vi "labview-traffic-light.vi"() -> ()   [LabVIEW 2022 SP3]
panel:
  out "Time":dbl
  in  "Yellow Time":dbl
  in  "Red Time":dbl
  in  "Green Time":dbl
  out "Red":bool
  out "yellow":bool
  out "Green":bool
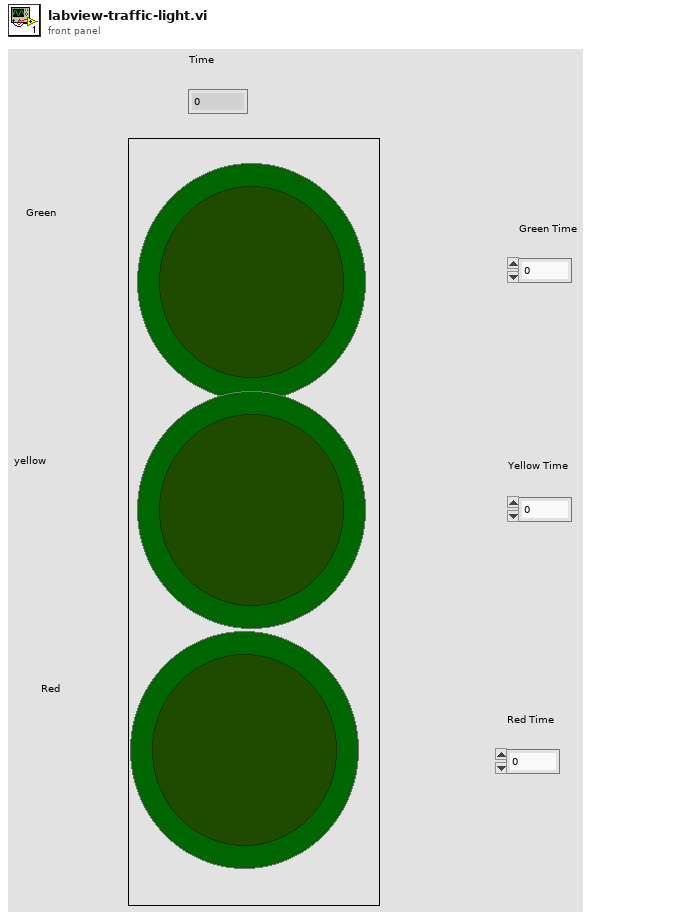
[diagram p1: front panel]
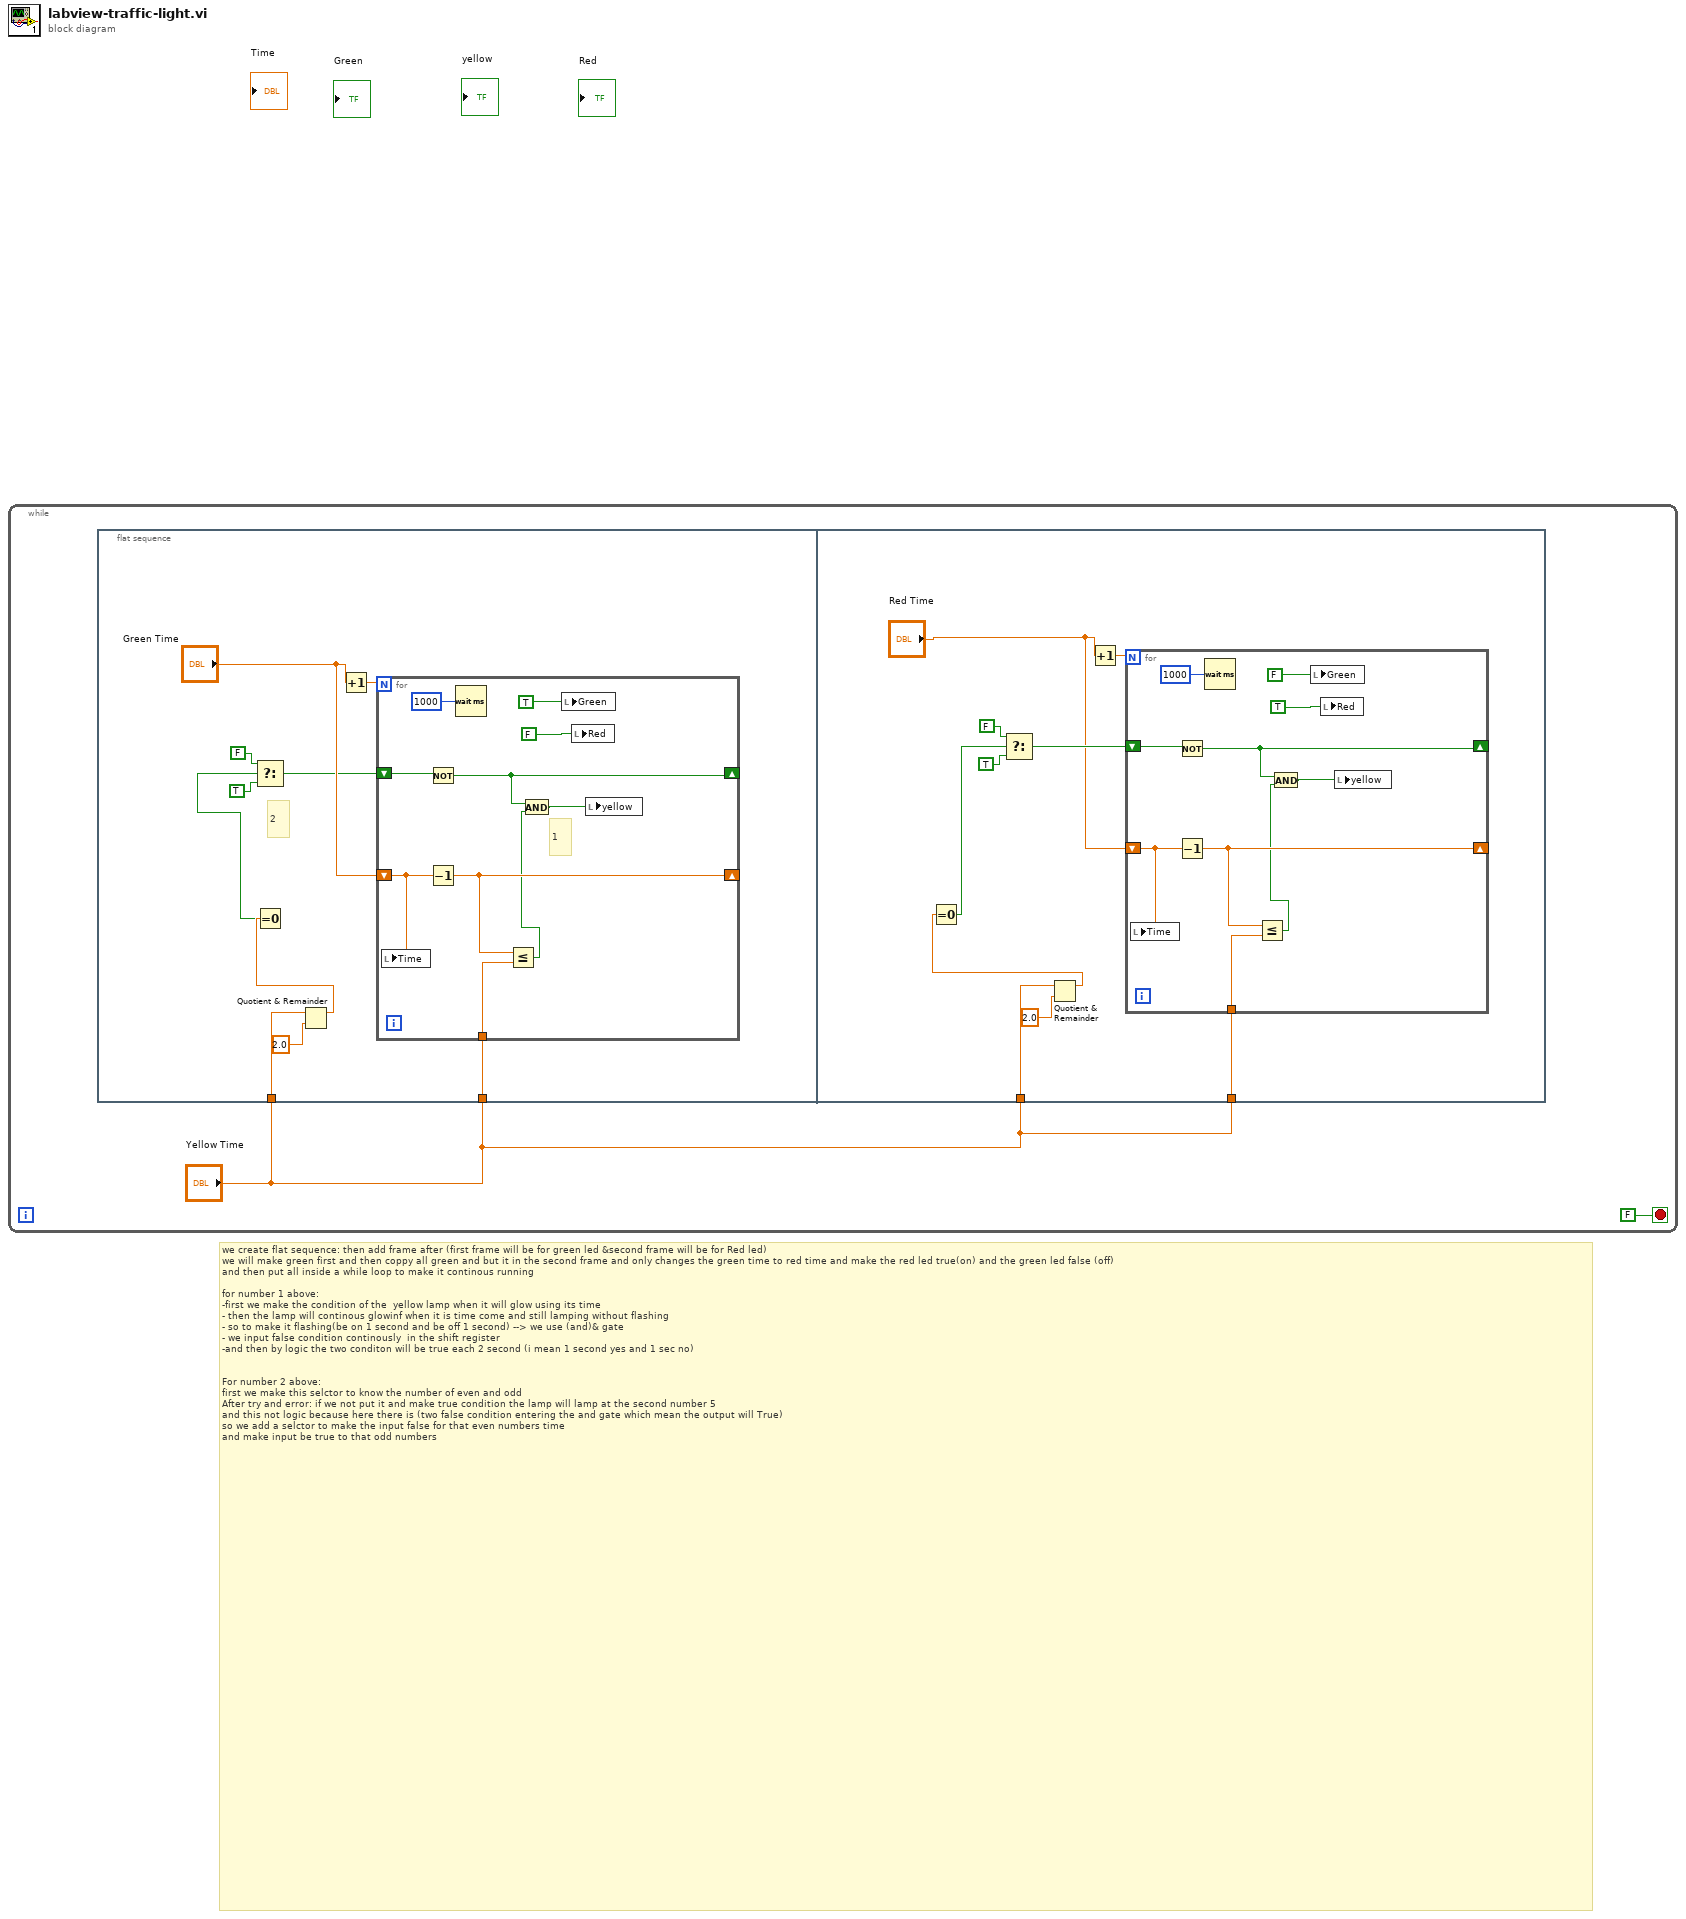
[diagram p0: block diagram]
diagram:
  # "we create flat sequence: then add frame after (first frame will be for green led &second frame will be for Red led)\nwe will make green first and then coppy all green and but it in the second frame and only changes the green time to red time and make the red led true(on) and the green led false (off) \nand then put all inside a while loop to make it continous running\n\nfor number 1 above:\n-first we make the condition of the  yellow lamp when it will glow using its time \n- then the lamp will continous glowinf when it is time come and still lamping without flashing\n- so to make it flashing(be on 1 second and be off 1 second) --> we use (and)& gate\n- we input false condition continously  in the shift register\n-and then by logic the two conditon will be true each 2 second (i mean 1 second yes and 1 sec no) \n\n\nFor number 2 above:\nfirst we make this selctor to know the number of even and odd\nAfter try and error: if we not put it and make true condition the lamp will lamp at the second number 5\nand this not logic because here there is (two false condition entering the and gate which mean the output will True)\nso we add a selctor to make the input false for that even numbers time \nand make input be true to that odd numbers"
  n1 = while {
    stop <- FALSE stop-if-true
    n2 = flat-sequence {
      tunnel: "Yellow Time" -> [w12]
      tunnel: "Yellow Time" -> [w8]
      tunnel: "Yellow Time" -> [w26]
      tunnel: "Yellow Time" -> [w25]
      frame #0 {
        # "2"
        n3 = Quotient & Remainder(x=w8, y=2.0) -> (x-y*floor(x/y)=w6:dbl)  [unwired: 1 out]
        n4 = Equal To 0?(x=w6) -> (x = 0?=w5:bool)
        n5 = Select(t=FALSE, s=w5, f=TRUE) -> (s? t:f=w9:bool)
        n6 = Increment(x="Green Time") -> (x+1=w11:dbl)
        n7 = for {
          N: w11 -> [_]
          shift-right: [w17] -> _
          shift-left: "Green Time" -> [w19]
          shift-right: [w15] -> _
          shift-left: w9 -> [w16]
          tunnel: w12 -> [w18]
          # "1"
          n8 = local write "Time"(w19) -> ()
          n9 = Not(x=w16) -> (.not. x?=w15:bool)
          n10 = Decrement(x=w19) -> (x-1=w17:dbl)
          n11 = Wait (ms)(milliseconds to wait=u32 1000) -> ()  [unwired: 1 out]
          n12 = Less Or Equal?(x=w17, y=w18) -> (x <= y?=w14:bool)
          n13 = And(x=w15, y=w14) -> (x .and. y?=w13:bool)
          n14 = local write "Green"(TRUE ("Green")) -> ()
          n15 = local write "Red"(FALSE ("Red")) -> ()
          n16 = local write "yellow"(w13) -> ()
        }
      }
      frame #1 {
        n17 = Quotient & Remainder(x=w26, y=2.0) -> (x-y*floor(x/y)=w29:dbl)  [unwired: 1 out]
        n18 = Equal To 0?(x=w29) -> (x = 0?=w23:bool)
        n19 = Select(t=FALSE, s=w23, f=TRUE) -> (s? t:f=w31:bool)
        n20 = Increment(x="Red Time") -> (x+1=w32:dbl)
        n21 = for {
          N: w32 -> [_]
          shift-right: [w37] -> _
          shift-left: "Red Time" -> [w39]
          shift-right: [w35] -> _
          shift-left: w31 -> [w36]
          tunnel: w25 -> [w38]
          n22 = local write "Time"(w39) -> ()
          n23 = Not(x=w36) -> (.not. x?=w35:bool)
          n24 = Decrement(x=w39) -> (x-1=w37:dbl)
          n25 = Wait (ms)(milliseconds to wait=u32 1000) -> ()  [unwired: 1 out]
          n26 = Less Or Equal?(x=w37, y=w38) -> (x <= y?=w34:bool)
          n27 = And(x=w35, y=w34) -> (x .and. y?=w33:bool)
          n28 = local write "Green"(FALSE ("Green")) -> ()
          n29 = local write "Red"(TRUE ("Red")) -> ()
          n30 = local write "yellow"(w33) -> ()
        }
      }
    }
  }
